vi "Channel Source Power Get Attenuation Auto.vi"(8 "error in (no error)":errorcluster {"code" format="%.0x"}, 9 "PortVal":i32 format="%.0g", 10 "RepCapIdentifier":string, 11 "instrument handle":refnum<k15>) -> (0 "error out":errorcluster {"code" format="%.0x"}, 2 "RetVal":bool, 3 "instrument handle out":refnum<k15>)   [LabVIEW 2014, in "Agilent NA.lvlib"]
doc: "Sets the Auto Attenuation value of the specified port"
uses:
  Agilent NA.lvlib
  AgNA.dll
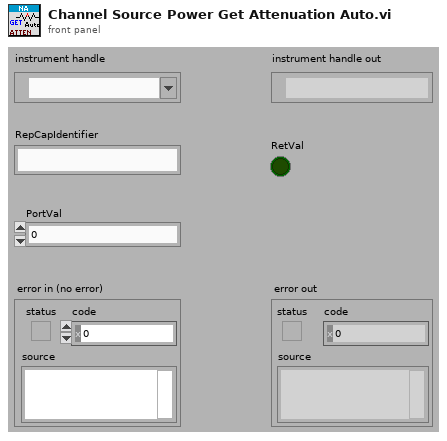
[diagram p1: front panel]
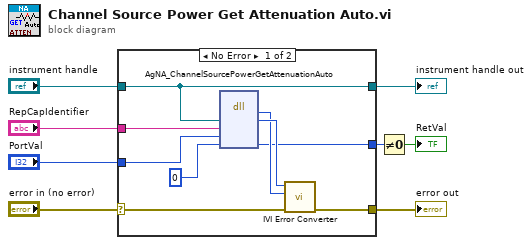
[diagram p0: block diagram]
diagram:
  n1 = case shown="No Error" "error in (no error)" {
    selector: "error in (no error)" -> [w15 w19]
    tunnel: [w14 w19] -> w8
    tunnel: "RepCapIdentifier" -> [w13 _]
    tunnel: "PortVal" -> [w12 _]
    tunnel: [w10 _] -> w3
    tunnel: [w9 w18] -> w2
    tunnel: "instrument handle" -> [w9 w18]
    frame No Error {
      n2 = dll-call lib="AgNA**.dll" fn="AgNA_ChannelSourcePowerGetAttenuationAuto"("Vi"=w9, "RepCapIdentifier"=w13, "PortVal"=w12, "RetVal"=i16 0) -> (w16:i32, "Vi"=w17:u32, "RetVal"=w10:i16)  [unwired: 5 in, 2 out]
      n3 = call "IVI Error Converter.vi"("error in (no error)"=w15, "IVI error code (0)"=w16, "instrument handle"=w17) -> ("error out"=w14:errorcluster)  [unwired: 7 in, 1 out]
    }
    frame Error {
    }
  }
  "error out" <- w8
  "instrument handle out" <- w2
  n4 = Not Equal To 0?(x=w3) -> (x != 0?=→"RetVal":bool)
